vi "Get Page ID.vi"(8 "Error In (No Error)":errorcluster, 9 "User Email":string="myemail", 10 "Notebook Name":string="My notebook on One Drive", 11 "client handle":T1) -> (0 "error out":errorcluster, 2 "Page ID":string, 3 "client handle out":T1)   [LabVIEW 2019, in "OneNote Library.lvlib"]
uses:
  OneNote Library.lvlib
  <vilib>/httpClient/ClientHandle.ctl
  <vilib>/JDP Science/JSONtext/String Subset.vi
  <vilib>/JDP Science/JSONtext/support/Strip Quotes and Unescape.vi
  <vilib>/JDP Science/JSONtext/support/Unescape JSON string.vi
  <vilib>/JDP Science/JSONtext/Parsing/Parse Full Path or Item Name.vi
  <vilib>/JDP Science/JSONtext/Offset/Find Item Locations by Path.vi
  Useful OAuth VIs/globals.vi
  <vilib>/httpClient/POSTBuffer.vi
  <vilib>/JDP Science/JSONtext/Next JSON Value.vi
  <vilib>/JDP Science/JSONtext/support/Error Cluster From Code.vi
  <vilib>/httpClient/LabVIEWHTTPClient.lvlib
  <vilib>/JDP Science/JSONtext/JSONtext.lvlib
  Useful HTTP VIs/Useful HTTP VIs.lvlib
  Useful OAuth VIs/Useful OAuth VIs.lvlib
panel:
  out "headers 2":string
  out "body 2":string
  out "Result":string
  out "date/time string":string
  out "LabVIEW TimeStamp":timestamp
  out "key not found?":bool
  out "map":map{string, string}(c390)
  out "Request URI":string caption="Result"
  out "body":string
  out "headers":string
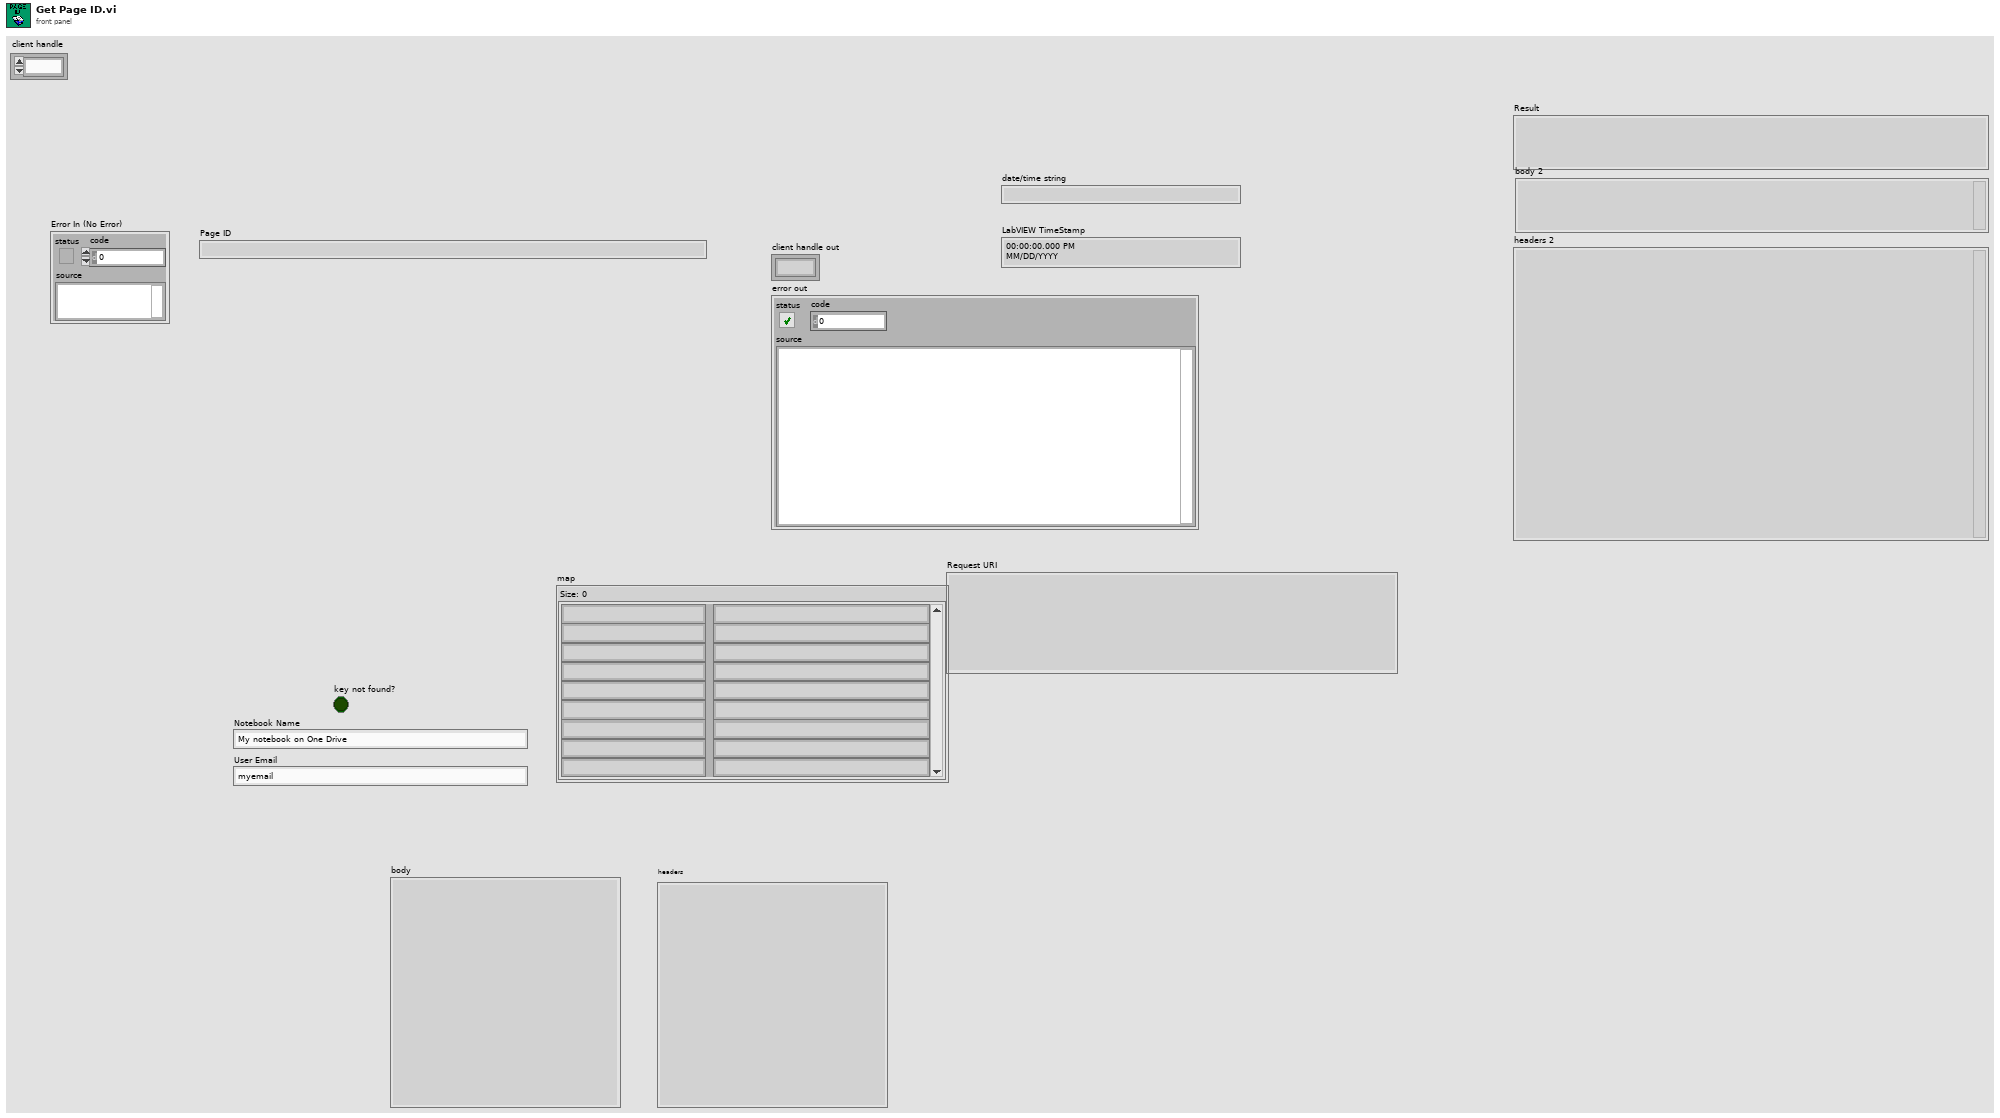
[diagram p1: front panel]
types:
  T1 = typedef "LabVIEWHTTPClient.lvlib/ClientHandle.ctl" = refnum<k1>
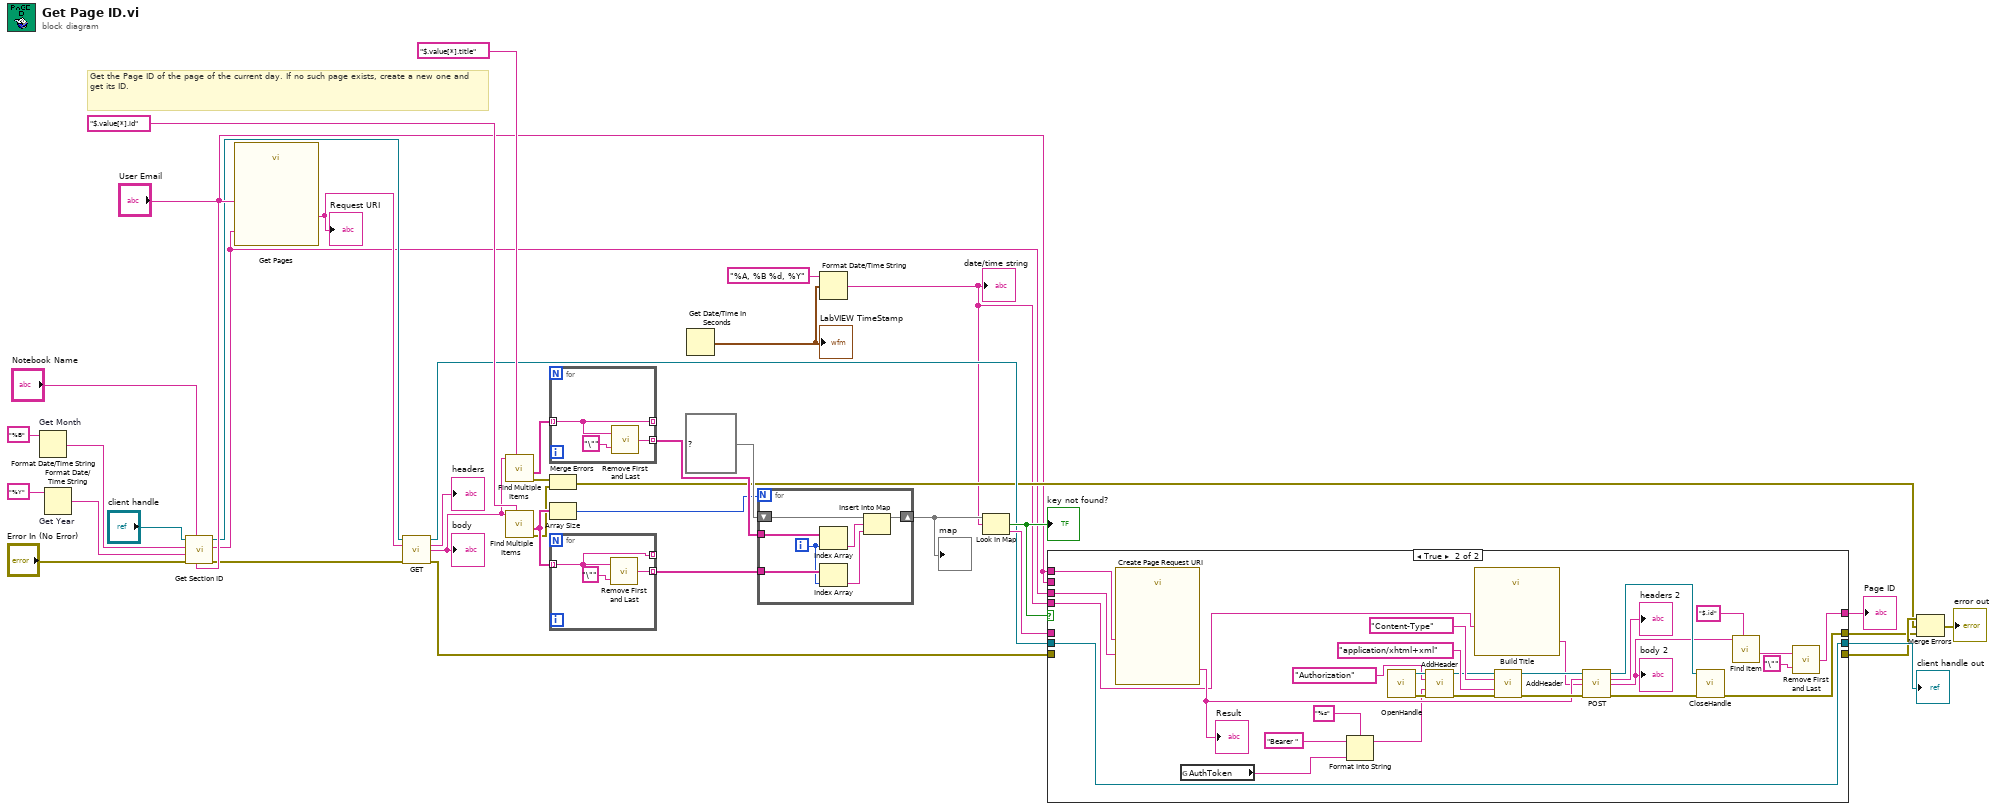
[diagram p0: block diagram]
diagram:
  # "Get the Page ID of the page of the current day. If no such page exists, create a new one and get its ID."
  n1 = Format Date/Time String "Get Month"(time format string (%c)="%B") -> (date/time string=w3:string)  [unwired: 2 in]
  n2 = Format Date/Time String "Get Year"(time format string (%c)="%Y") -> (date/time string=w4:string)  [unwired: 2 in]
  n3 = call "Get Section ID.vi"("User Email"="User Email", "Notebook Name"="Notebook Name", "Error In (No Error)"="Error In (No Error)", "Year (Section Group)"=w4, "Month (Section)"=w3, "client handle"="client handle") -> ("error out"=w6:errorcluster, "Section ID"=w5:string, "client handle out"=w7:T1)  [unwired: 3 in]
  n4 = call "Get Pages"("user"="User Email", "Section ID"=w5) -> ("Result"=w38:string)  [unwired: 12 in, 1 out]
  "Request URI" <- w38
  n5 = call <vilib>:"GET.vi"("client handle"=w7, "url"=w38, "error in (no error)"=w6) -> ("client handle out"=w23:T1, "headers"=→"headers":string, "body"=w35:string, "error out"=w21:errorcluster)  [unwired: 9 in]
  "body" <- w35
  n6 = call <vilib>:"Find Multiple Items.vi"("$Path or Item Name"="$.value[*].title", "JSON"=w35) -> ("error out"=w20:errorcluster, "<JSON>"=w33:string[])  [unwired: 6 in, 2 out]
  n7 = call <vilib>:"Find Multiple Items.vi"("$Path or Item Name"="$.value[*].id", "JSON"=w35) -> ("error out"=w19:errorcluster, "<JSON>"=w29:string[])  [unwired: 6 in, 2 out]
  n8 = for {
    tunnel: w33 -> [w39] mode=indexing
    tunnel: [w39] -> _ mode=indexing
    tunnel: [w40] -> w32 mode=indexing
    n9 = call "Remove First and Last.vi"("Char to Remove"="\"", "String"=w39) -> ("Result"=w40:string)
  }
  n10 = Merge Errors(w20, w19) -> (w17:errorcluster)
  n11 = Array Size(array=w29) -> (size(s)=w28:i32)
  n12 = for {
    tunnel: w29 -> [w42] mode=indexing
    tunnel: [w42] -> _ mode=indexing
    tunnel: [w43] -> w31 mode=indexing
    n13 = call "Remove First and Last.vi"("Char to Remove"="\"", "String"=w42) -> ("Result"=w43:string)
  }
  n14 = Get Date/Time In Seconds() -> (seconds since 1Jan1904=w12:timestamp)
  "LabVIEW TimeStamp" <- w12
  n15 = for {
    N: w28 -> [_]
    tunnel: w31 -> [w51]
    tunnel: w32 -> [w50]
    shift-right: [w47] -> w27
    shift-left: map{string, string} {} ("map") -> [w49]
    i -> [w48]
    n16 = Index Array(array=w50, index=w48) -> (element=w46:string)
    n17 = Index Array(array=w51, index=w48) -> (element=w45:string)
    n18 = Insert Into Map(map in=w49, key=w46, value=w45) -> (map out=w47:map{string, string})  [unwired: 2 out]
  }
  "map" <- w27
  n19 = Format Date/Time String(time format string (%c)="%A, %B %d, %Y", seconds (now)=w12) -> (date/time string=w8:string)  [unwired: 1 in]
  "date/time string" <- w8
  n20 = Look In Map(map=w27, key=w8) -> (key not found?=w26:bool, value=w25:string)  [unwired: 1 in]
  "key not found?" <- w26
  n21 = case shown="True" w26 {
    tunnel: "User Email" -> [_ _]
    tunnel: w25 -> [w54 _]
    tunnel: [w54 w66] -> w24
    tunnel: [w52 _] -> w18
    tunnel: w23 -> [w53 w82]
    tunnel: [w53 w82] -> w22
    tunnel: w21 -> [w52 _]
    tunnel: w8 -> [_ w72]
    tunnel: "User Email" -> [_ w71]
    tunnel: w5 -> [_ w65]
    tunnel: [_ w64] -> w2
    frame False {
    }
    frame True {
      n22 = call "Create Page Request URI"("user email"=w71, "Section ID"=w65) -> ("Result"=w77:string)  [unwired: 12 in, 1 out]
      "Result" <- w77
      n23 = global read "globals.vi" "AuthToken"() -> (w56:string)
      n24 = Format Into String(format string="%s", initial string="Bearer ", w56) -> (resulting string=w55:string)  [unwired: 1 in, 1 out]
      n25 = call <vilib>:"OpenHandle.vi"() -> ("client handle out"=w63:T1, "error out"=w62:errorcluster)  [unwired: 14 in]
      n26 = call <vilib>:"AddHeader.vi"("client handle"=w63, "header"="Authorization", "value"=w55, "error in (no error)"=w62) -> ("client handle out"=w59:T1, "error out"=w61:errorcluster)  [unwired: 10 in]
      n27 = call "Build Title"("Title"=w72) -> ("Result"=w76:string)  [unwired: 13 in, 1 out]
      n28 = call <vilib>:"AddHeader.vi"("client handle"=w59, "header"="Content-Type", "value"="application/xhtml+xml", "error in (no error)"=w61) -> ("client handle out"=w79:T1, "error out"=w78:errorcluster)  [unwired: 10 in]
      n29 = call-poly <vilib>:"POST.vi"("client handle"=w79, "url"=w77, "buffer"=w76, "error in (no error)"=w78) -> ("client handle out"=w74:T1, "headers"=→"headers 2":string, "body"=w70:string, "error out"=w73:errorcluster)  [unwired: 8 in]
      "body 2" <- w70
      n30 = call <vilib>:"CloseHandle.vi"("client handle"=w74, "error in (no error)"=w73) -> ("error out"=w64:errorcluster)  [unwired: 13 in]
      n31 = call <vilib>:"Find Item.vi"("$Path or Item Name"="$.id", "JSON"=w70) -> ("<JSON>"=w68:string)  [unwired: 6 in, 3 out]
      n32 = call "Remove First and Last.vi"("Char to Remove"="\"", "String"=w68) -> ("Result"=w66:string)
    }
  }
  "Page ID" <- w24
  "client handle out" <- w22
  n33 = Merge Errors(w18, w17, w2) -> (→"error out":errorcluster)
